vi "Close Logger.vi"(8 "error in (no error)":errorcluster, 11 "Logger in.lvclass":refnum<class "Logger.lvclass">) -> (0 "error out":errorcluster)   [LabVIEW 2021, in "Logger.lvclass"]
uses:
  Logger.lvclass
  Logger.lvclass/Logger.ctl
  <vilib>/Skyline/Tag/Wrapper/Wrapper_class/Close Tag (Single).vi
  <vilib>/Skyline/Message/HTTP Wrapper/NI Skyline Message HTTP.lvclass
  <vilib>/Skyline/Tag/Wrapper/Wrapper_class/NI Skyline Tag.lvclass
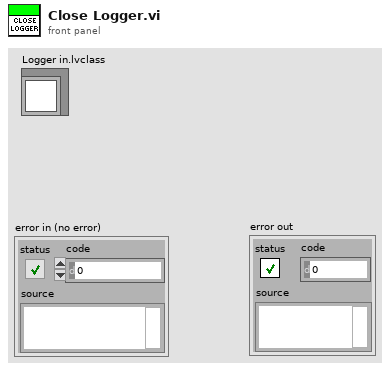
[diagram p1: front panel]
types:
  T1 = cluster{"Tag Units":string, "Tag Path":string, "Tag Reference":refnum<class "NI Skyline Tag.lvclass">}[]
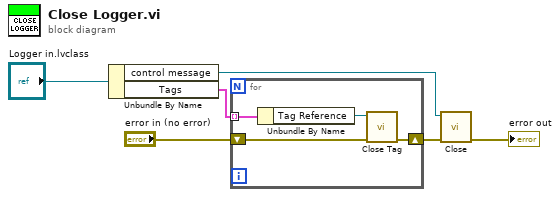
[diagram p0: block diagram]
diagram:
  n1 = Unbundle By Name("Logger in.lvclass") -> ("control message"=w2:refnum<class "NI Skyline Message HTTP.lvclass">, "Tags"=w1:T1)
  n2 = for {
    tunnel: w1 -> [w10] mode=indexing
    shift-right: [w8] -> w3
    shift-left: "error in (no error)" -> [w9]
    n3 = Unbundle By Name(w10) -> ("Tag Reference"=w7:refnum<class "NI Skyline Tag.lvclass">)
    n4 = call-poly <vilib>:"Close Tag.vi"("error in (no error)"=w9, "tag"=w7) -> ("error out"=w8:errorcluster)  [unwired: 9 in]
  }
  n5 = call-dynamic "Close.vi"("error in (no error)"=w3, "message session"=w2) -> ("error out"=→"error out":errorcluster)  [unwired: 9 in]
